vi "Main.vi"(11 "Error In":errorcluster) -> (15 "Error Out":errorcluster)   [LabVIEW 2023]
doc: "The VI is a launcher VI that allows to perform the sender to receiver communication"
uses:
  Controls/Queue Operation.ctl
  Controls/User Event Operations.ctl
  Controls/Launcher Data.ctl
  Controls/VI reference.ctl
  Classes/Sender/Methods/Sender UI.vi
  Classes/Receiver/Methods/Receiver UI.vi
  Classes/Sender/Sender.lvclass
  Classes/Receiver/Receiver.lvclass
panel:
  # "Instructions:\n1. Run the VI.\n2. View the sender and receiver loaded in the front panel.\n3. Select the transmission data type.\n4. Click the notify button to send notification to the receiver.\n5. Click notify with data to send one data at a time.\n6. Click stream data to continuously stream data to the receiver and click stop stream to stop.\n7. Click panel close to stop the VI running"
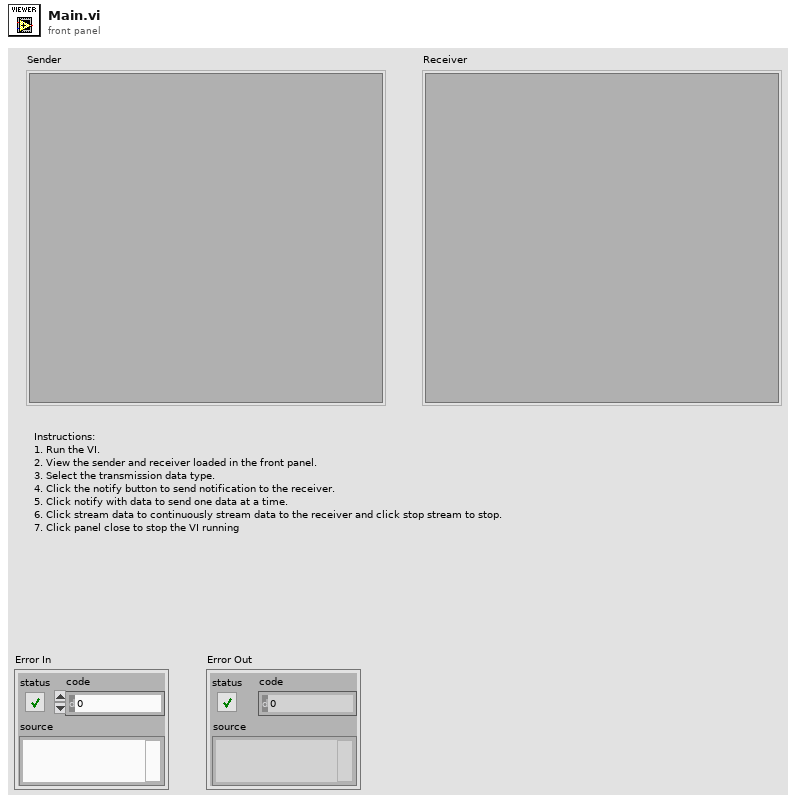
[diagram p1: front panel]
types:
  T1 = typedef "Launcher Data.ctl" = cluster{"Sender Clones":string[], "Sender Clone Number":i32, "Receiver Clones":string[], "Receiver Clone Number":i32, "Tag":string, "VI ref Array":T2[], "Active Sender Ref":refnum<vi>, "Active Receiver Ref":refnum<vi>}
  T2 = typedef "VI reference.ctl" = cluster{"Tag":string, "VI Refnum":refnum<vi>}
  T3 = typedef "User Event Operations.ctl" = enum16{"Obtain", "Generate", "Destroy"}
  T4 = typedef "Queue Operation.ctl" = enum16{"Create & Enqueue N", "Enqueue N", "Dequeue", "Enstack N", "Flush", "Release"}
  T5 = typedef "Queue Element.ctl" = cluster{"State":string, "Data":variant}
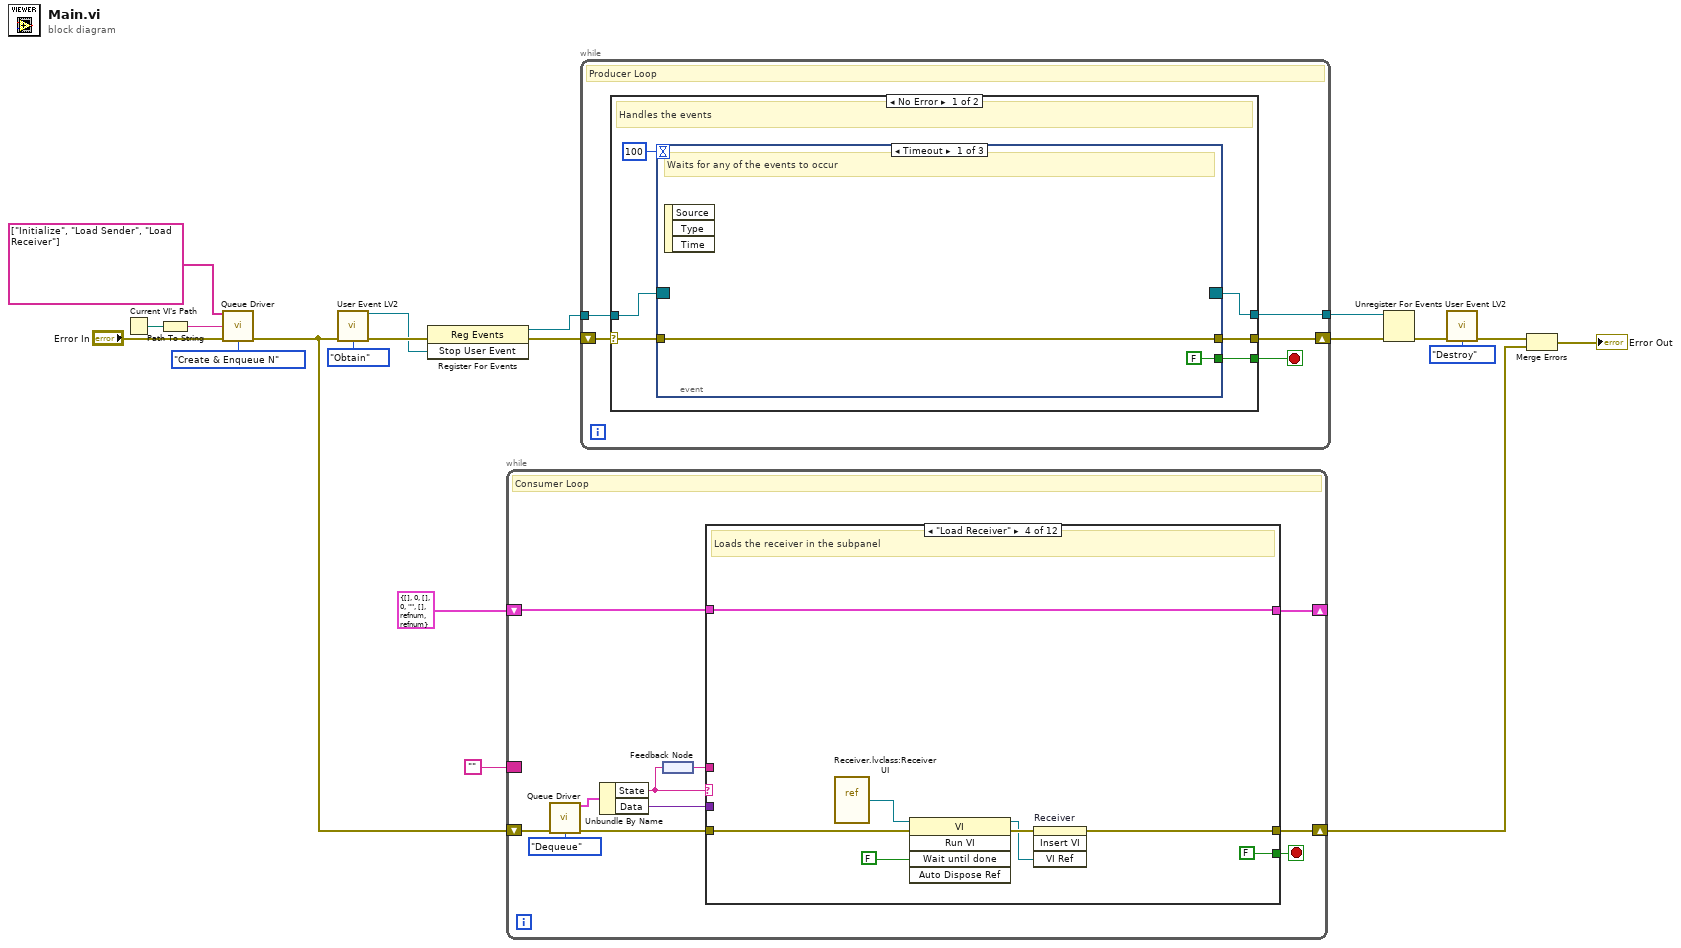
[diagram p0: block diagram]
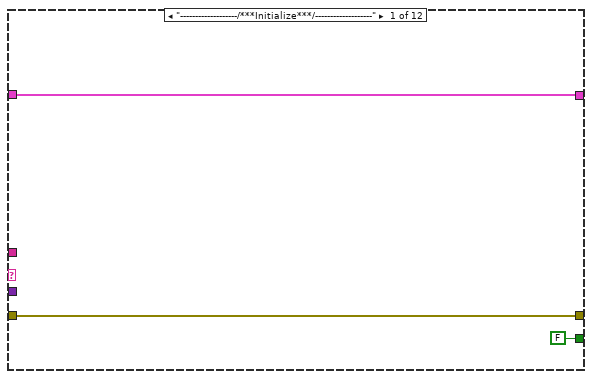
[diagram p2: hidden frame]
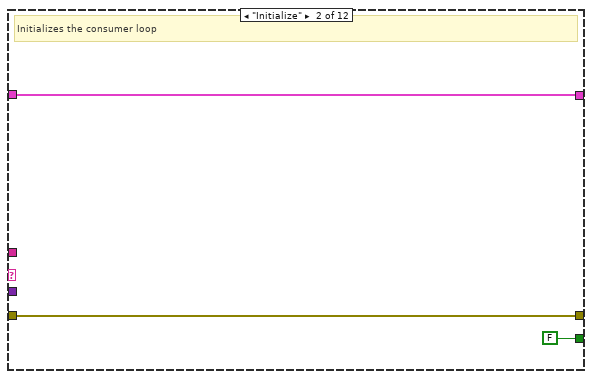
[diagram p3: hidden frame]
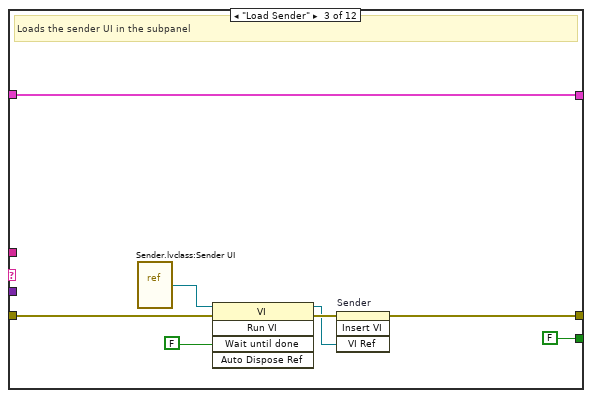
[diagram p4: hidden frame]
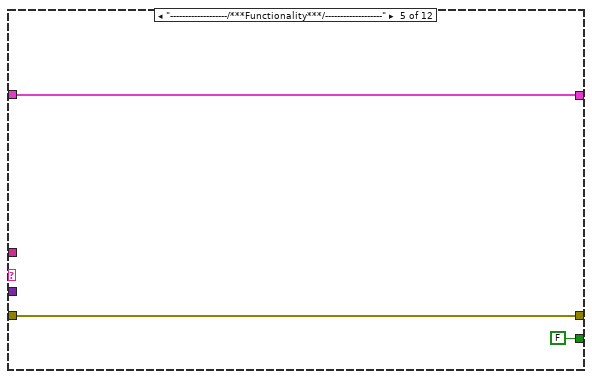
[diagram p5: hidden frame]
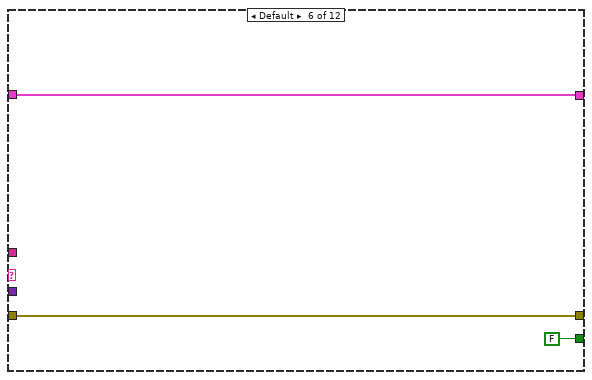
[diagram p6: hidden frame]
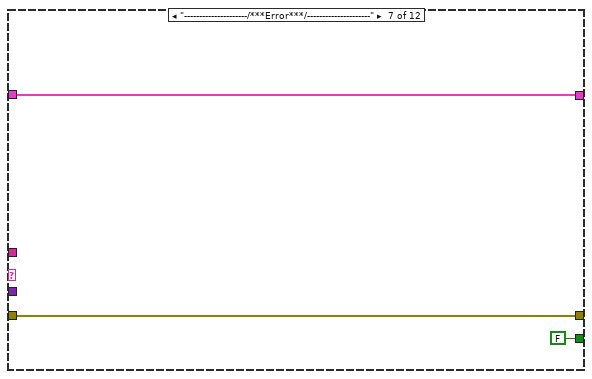
[diagram p7: hidden frame]
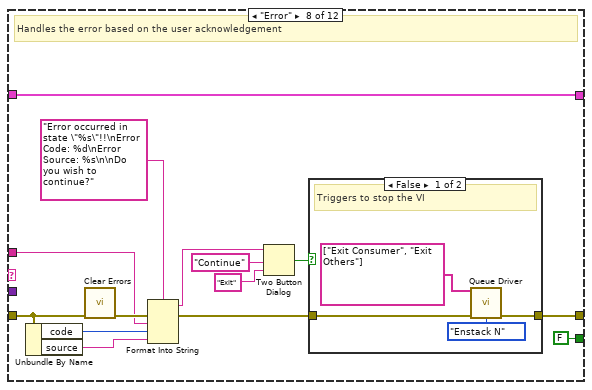
[diagram p8: hidden frame]
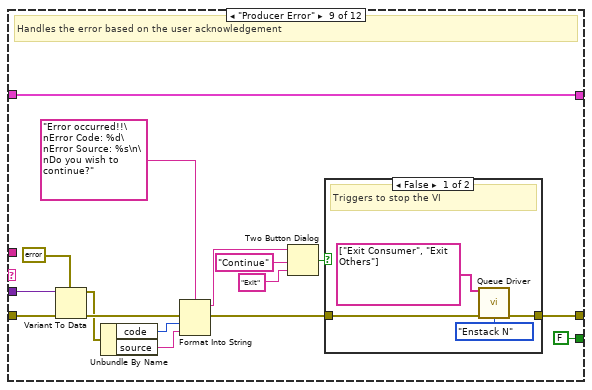
[diagram p10: hidden frame]
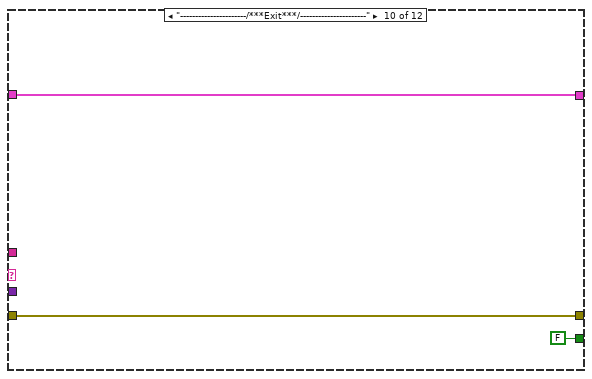
[diagram p12: hidden frame]
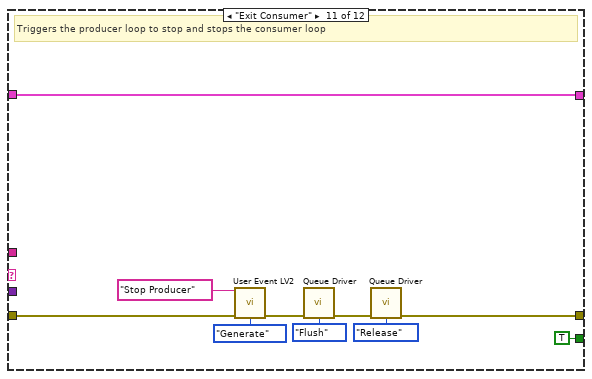
[diagram p13: hidden frame]
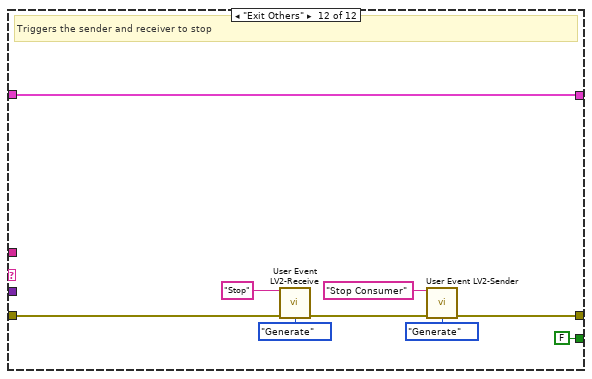
[diagram p14: hidden frame]
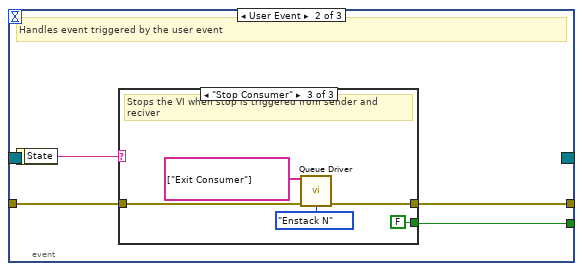
[diagram p15: hidden frame]
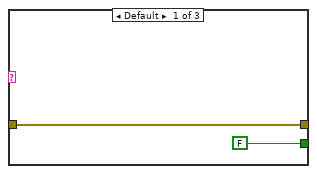
[diagram p16: hidden frame]
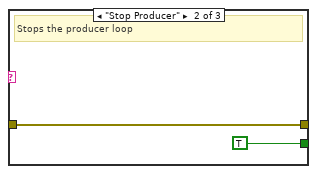
[diagram p17: hidden frame]
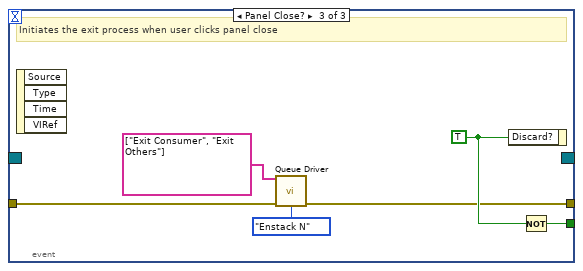
[diagram p18: hidden frame]
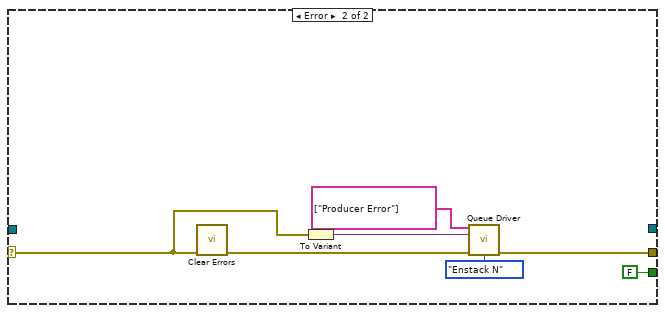
[diagram p19: hidden frame]
diagram:
  n1 = Current VI's Path() -> (path=w17:path)
  n2 = Path To String(path=w17) -> (string=w1:string)
  n3 = call "Queue Driver.vi"("States[]"=string[] ["Initialize", "Load Sender", "Load Receiver"], "Queue Name"=w1, "Error In"="Error In", "Queue Operation"=Queue_Operation."Create & Enqueue N") -> ("Error Out"=w11:errorcluster)  [unwired: 10 in, 1 out]
  n4 = call "User Event LV2.vi"("Error In"=w11, "Operation"=User_Event_Operations."Obtain") -> ("Stop User Event"=w9:refnum<user-event>, "Error Out"=w13:errorcluster)  [unwired: 12 in]
  n5 = register-events(error in=w13, w9) -> (reference out=w8:refnum<event-registration>, error out=w10:errorcluster)  [unwired: 1 in]
  n6 = while {
    shift-right: [w30] -> w14
    shift-left: w11 -> [w31]
    border: "" -> [_]
    shift-right: [w23] -> _
    shift-left: T1 {"Sender Clones"=[], "Sender Clone Number"=0, "Receiver Clones"=[], "Receiver Clone Number"=0, "Tag"="", "VI ref Array"=[], "Active Sender Ref"=refnum, "Active Receiver Ref"=refnum} -> [w24]
    stop <- w27 stop-if-true
    # "Consumer Loop"
    n7 = call "Queue Driver.vi"("Error In"=w31, "Queue Operation"=Queue_Operation."Dequeue") -> ("Dequeue Element"=w21:T5, "Error Out"=w29:errorcluster)  [unwired: 12 in]
    n8 = Unbundle By Name(w21) -> ("State"=w26:string, "Data"=w22:variant)
    n9 = feedback-in #1(w26) -> ()
    n10 = feedback #1() -> (w25:string)
    n11 = case shown="\"Load Receiver\"" w26 {
      tunnel: w29 -> [w34 w37 w45 w53 w56 w59 w62 w68 w92 w105 w115 w124]
      tunnel: [w34 w37 w39 w47 w56 w59 w62 w65 w90 w105 w111 w118] -> w30
      tunnel: [FALSE FALSE FALSE FALSE FALSE FALSE FALSE FALSE FALSE FALSE TRUE FALSE] -> w27
      tunnel: w25 -> [_ _ _ _ _ _ _ w66 _ _ _ _]
      tunnel: w24 -> [w32 w35 w43 w51 w54 w57 w60 w63 w88 w103 w106 w122]
      tunnel: [w32 w35 w43 w51 w54 w57 w60 w63 w88 w103 w106 w122] -> w23
      tunnel: w22 -> [_ _ _ _ _ _ _ _ w87 _ _ _]
      frame "-------------------/***Initialize***/-------------------" {
      }
      frame "Initialize" {
        # "Initializes the consumer loop"
      }
      frame "Load Sender" {
        # "Loads the sender UI in the subpanel"
        n12 = vi-ref "Sender.lvclass:Sender UI.vi"() -> (w41:refnum<vi>)
        n13 = invoke class="VI" method="Run VI"(reference=w41, error in=w45, "Wait until done"=FALSE ("Wait Until Done")) -> (reference out=w38:refnum<vi>, error out=w42:errorcluster)  [unwired: 2 in, 3 out]
        n14 = invoke on="Sender" class="SubPnl" method="Insert VI"(error in=w42, "VI Ref"=w38) -> (error out=w39:errorcluster)  [unwired: 2 in, 3 out]
      }
      frame "Load Receiver" {
        # "Loads the receiver in the subpanel"
        n15 = vi-ref "Receiver.lvclass:Receiver UI.vi"() -> (w49:refnum<vi>)
        n16 = invoke class="VI" method="Run VI"(reference=w49, error in=w53, "Wait until done"=FALSE ("Wait Until Done")) -> (reference out=w46:refnum<vi>, error out=w50:errorcluster)  [unwired: 2 in, 3 out]
        n17 = invoke on="Receiver" class="SubPnl" method="Insert VI"(error in=w50, "VI Ref"=w46) -> (error out=w47:errorcluster)  [unwired: 2 in, 3 out]
      }
      frame "-------------------/***Functionality***/-------------------" {
      }
      frame Default {
      }
      frame "---------------------/***Error***/---------------------" {
      }
      frame "Error" {
        # "Handles the error based on the user acknowledgement"
        n18 = Unbundle By Name(w68) -> ("code"=w70:i32, "source"=w69:string)
        n19 = call <vilib>:"Clear Errors.vi"("error in (no error)"=w68) -> ("error out"=w75:errorcluster)  [unwired: 5 in, 1 out]
        n20 = Format Into String(format string="Error occurred in state \"%s\"!!\nError Code: %d\nError Source: %s\n\nDo you wish to continue?", error in=w75, w66, w70, w69) -> (resulting string=w73:string, error out=w67:errorcluster)  [unwired: 1 in]
        n21 = Two Button Dialog(message=w73, 1:"Exit" ("F button name (\"Cancel\")"), 2:"Continue" ("T button name (\"OK\")")) -> (T button?=w64:bool)
        n22 = case shown="False" w64 {
          tunnel: w67 -> [w80 w81]
          tunnel: [w79 w81] -> w65
          frame False {
            # "Triggers to stop the VI"
            n23 = call "Queue Driver.vi"("States[]"=string[] ["Exit Consumer", "Exit Others"], "Error In"=w80, "Queue Operation"=Queue_Operation."Enstack N") -> ("Error Out"=w79:errorcluster)  [unwired: 11 in, 1 out]
          }
          frame True {
          }
        }
      }
      frame "Producer Error" {
        # "Handles the error based on the user acknowledgement"
        n24 = Variant To Data(error in=w92, type=errorcluster {"status"=FALSE, "code"=0, "source"=""} ("error out"), Variant=w87) -> (data=w84:errorcluster, error out=w86:errorcluster)
        n25 = Unbundle By Name(w84) -> ("code"=w83:i32, "source"=w82:string)
        n26 = Format Into String(format string="Error occurred!!\nError Code: %d\nError Source: %s\n\nDo you wish to continue?", error in=w86, w83, w82) -> (resulting string=w95:string, error out=w91:errorcluster)  [unwired: 1 in]
        n27 = Two Button Dialog(message=w95, 1:"Exit" ("F button name (\"Cancel\")"), 2:"Continue" ("T button name (\"OK\")")) -> (T button?=w89:bool)
        n28 = case shown="False" w89 {
          tunnel: w91 -> [w101 w102]
          tunnel: [w100 w102] -> w90
          frame False {
            # "Triggers to stop the VI"
            n29 = call "Queue Driver.vi"("States[]"=string[] ["Exit Consumer", "Exit Others"], "Error In"=w101, "Queue Operation"=Queue_Operation."Enstack N") -> ("Error Out"=w100:errorcluster)  [unwired: 11 in, 1 out]
          }
          frame True {
          }
        }
      }
      frame "----------------------/***Exit***/----------------------" {
      }
      frame "Exit Consumer" {
        # "Triggers the producer loop to stop and stops the consumer loop"
        n30 = call "User Event LV2.vi"("Event Name"="Stop Producer", "Error In"=w115, "Operation"=User_Event_Operations."Generate") -> ("Error Out"=w109:errorcluster)  [unwired: 11 in, 1 out]
        n31 = call "Queue Driver.vi"("Error In"=w109, "Queue Operation"=Queue_Operation."Flush") -> ("Error Out"=w113:errorcluster)  [unwired: 12 in, 1 out]
        n32 = call "Queue Driver.vi"("Error In"=w113, "Queue Operation"=Queue_Operation."Release") -> ("Error Out"=w111:errorcluster)  [unwired: 12 in, 1 out]
      }
      frame "Exit Others" {
        # "Triggers the sender and receiver to stop"
        n33 = call "User Event LV2-Receive.vi"("Event Name"="Stop", "Error In"=w124, "Operation"=User_Event_Operations."Generate") -> ("Error Out"=w121:errorcluster)  [unwired: 11 in, 1 out]
        n34 = call "User Event LV2-Sender.vi"("Event Name"="Stop Consumer", "Error In"=w121, "Operation"=User_Event_Operations."Generate") -> ("Error Out"=w118:errorcluster)  [unwired: 11 in, 1 out]
      }
    }
  }
  n35 = while {
    shift-right: [w127] -> w19
    shift-left: w10 -> [w128]
    tunnel: w8 -> [w126]
    tunnel: [w125] -> w6
    stop <- w129 stop-if-true
    # "Producer Loop"
    n36 = case shown="No Error" w128 {
      selector: w128 -> [w134 w158]
      tunnel: [w135 FALSE] -> w129
      tunnel: [w133 w161] -> w127
      tunnel: w126 -> [w131 _]
      tunnel: [w130 _] -> w125
      frame No Error {
        # "Handles the events"
        n37 = event shown="[0] Timeout" {
          selector: w131 -> [_ _ _]
          dyn-events: [_ _ _] -> w130
          timeout: 100 -> [_ _ _]
          tunnel: [FALSE w138 w155] -> w135
          tunnel: w134 -> [w136 w141 w154]
          tunnel: [w136 w140 w153] -> w133
          event Timeout {
            # "Waits for any of the events to occur"
            n38 = event-data() -> ()  [unwired: 1 in, 3 out]
          }
          event User Event {
            # "Handles event triggered by the user event"
            n39 = event-data() -> ("State"=w139:string)  [unwired: 1 in]
            n40 = case shown="\"Stop Consumer\"" w139 {
              tunnel: w141 -> [w143 w145 w150]
              tunnel: [w143 w145 w148] -> w140
              tunnel: [FALSE TRUE FALSE] -> w138
              frame Default {
              }
              frame "Stop Producer" {
                # "Stops the producer loop"
              }
              frame "Stop Consumer" {
                # "Stops the VI when stop is triggered from sender and reciver"
                n41 = call "Queue Driver.vi"("States[]"=string[] ["Exit Consumer"], "Error In"=w150, "Queue Operation"=Queue_Operation."Enstack N") -> ("Error Out"=w148:errorcluster)  [unwired: 11 in, 1 out]
              }
            }
          }
          event Panel Close? {
            w156 = TRUE ("Discard?")
            # "Initiates the exit process when user clicks panel close"
            n42 = event-data() -> ()  [unwired: 1 in, 4 out]
            n43 = call "Queue Driver.vi"("States[]"=string[] ["Exit Consumer", "Exit Others"], "Error In"=w154, "Queue Operation"=Queue_Operation."Enstack N") -> ("Error Out"=w153:errorcluster)  [unwired: 11 in, 1 out]
            n44 = event-data("Discard?"=w156) -> ()  [unwired: 1 in, 1 out]
            n45 = Not(x=w156) -> (.not. x?=w155:bool)
          }
        }
      }
      frame Error {
        n46 = call <vilib>:"Clear Errors.vi"("error in (no error)"=w158) -> ("error out"=w162:errorcluster)  [unwired: 5 in, 1 out]
        n47 = To Variant(anything=w158) -> (Variant=w157:variant)
        n48 = call "Queue Driver.vi"("States[]"=string[] ["Producer Error"], "Data"=w157, "Error In"=w162, "Queue Operation"=Queue_Operation."Enstack N") -> ("Error Out"=w161:errorcluster)  [unwired: 10 in, 1 out]
      }
    }
  }
  n49 = Unregister For Events(event registration refnum=w6, error in=w19) -> (error out=w7:errorcluster)
  n50 = call "User Event LV2.vi"("Error In"=w7, "Operation"=User_Event_Operations."Destroy") -> ("Error Out"=w5:errorcluster)  [unwired: 12 in, 1 out]
  n51 = Merge Errors(w5, w14) -> (→"Error Out":errorcluster)
